vi "LinearSystemId_CreateSingleJointedArmSystem.vi"(9 "G":dbl, 10 "jKgSquaredMeters":dbl, 11 "DCMOTOR":T1 {"Jr_KgM2" format="%13.5p"; "L_H" format="%13.5p"; "Kt_NMPerAmp" format="%13.5p"; "KvINV_RadPerSecPerVolt" format="%13.5p"; "R_Ohms" format="%13.5p"; "FreeSpeed_RadPerSec" format="%13.5p"; "FreeCurrent_Amps" format="%13.5p"; "StallCurrent_Amps" format="%13.5p"; "StallTorque_NM" format="%13.5p"; "nominalVoltage_Volts" format="%13.5p"}) -> (0 "Size Coerced":bool, 3 "Linearsystem":T2)   [LabVIEW 2019, in "Trajectory_Library.lvlib"]
doc: "Create a state-space model of a single jointed arm system. The states of the system are [angle, angular velocity], inputs are [voltage], and outputs are [angle].\n\nInputs: \n - motor -- The motor (or gearbox) attached to the arm.\n - jKgSquaredMeters -- The moment of inertia J of the arm.\n - G -- The gearing between the motor and arm, in output over input. Most of the time this will be greater than 1.\n\nOutputs:\n - LinearSystem -- A LinearSystem representing the given characterized constants.\n - Error -- A boolean indicating an error occured creating the system. A value of TRUE indicates an error."
uses:
  Trajectory_Library.lvlib
  LINEAR_SYSTEM.ctl
  <vilib>/Analysis/Matrix/Datatypes/RealMatrix.ctl
  DCMOTOR.CTL
  <vilib>/Analysis/Matrix/NI_Matrix.lvlib
panel:
  # "<States,States>"
  # "<States,Inputs>"
  # "<Outputs,States>"
  # "<Outputs,Inputs>"
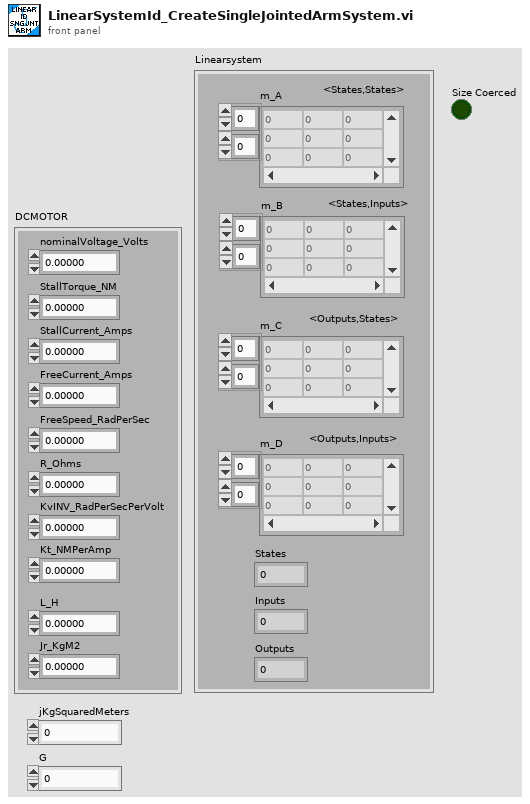
[diagram p1: front panel]
types:
  T1 = typedef "Trajectory_Library.lvlib/DCMOTOR.CTL" = cluster{"nominalVoltage_Volts":dbl, "StallTorque_NM":dbl, "StallCurrent_Amps":dbl, "FreeCurrent_Amps":dbl, "FreeSpeed_RadPerSec":dbl, "R_Ohms":dbl, "KvINV_RadPerSecPerVolt":dbl, "Kt_NMPerAmp":dbl, "L_H":dbl, "Jr_KgM2":dbl}
  T2 = typedef "Trajectory_Library.lvlib/LINEAR_SYSTEM.ctl" = cluster{"m_A":T3, "m_B":T3, "m_C":T3, "m_D":T3, "States":i32, "Inputs":i32, "Outputs":i32}
  T3 = typedef "NI_Matrix.lvlib/RealMatrix.ctl" = dbl[][]
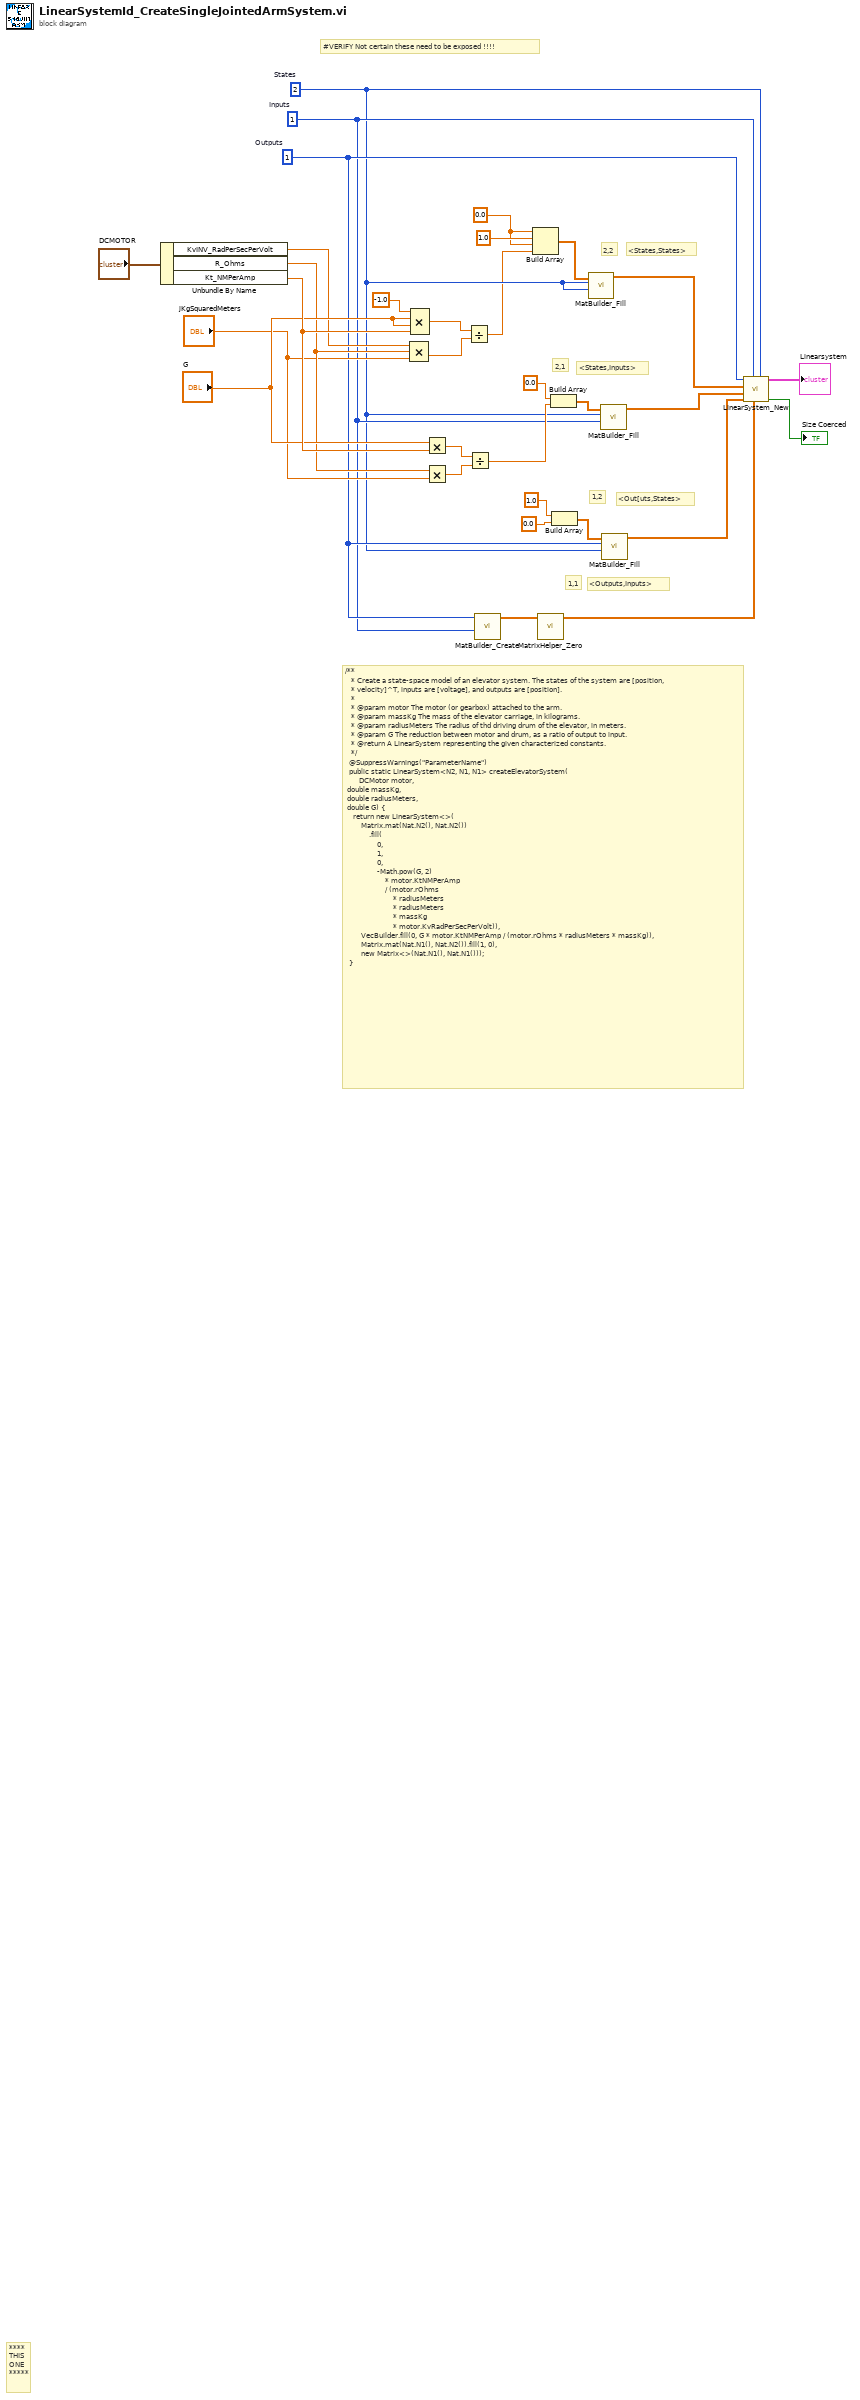
[diagram p0: block diagram]
diagram:
  w16 = 1  # Outputs
  w10 = 1  # Inputs
  w6 = 2  # States
  w4 = 0.0 ("element")
  # "2,2"
  # "2,1"
  # "1,2"
  # "1,1"
  # "<States,States>"
  # "<States,Inputs>"
  # "<Out[uts,States>"
  # "<Outputs,Inputs>"
  # "#VERIFY Not certain these need to be exposed !!!!"
  # "/**\n   * Create a state-space model of an elevator system. The states of the system are [position,\n   * velocity]^T, inputs are [voltage], and outputs are [position].\n   *\n   * @param motor The motor (or gearbox) attached to the arm.\n   * @param massKg The mass of the elevator carriage, in kilograms.\n   * @param radiusMeters The radius of thd driving drum of the elevator, in meters.\n   * @param G The reduction between motor and drum, as a ratio of output to input.\n   * @return A LinearSystem representing the given characterized constants.\n   */\n  @SuppressWarnings(\"ParameterName\")\n  public static LinearSystem<N2, N1, N1> createElevatorSystem(\n      \tDCMotor motor, \n\tdouble massKg, \n\tdouble radiusMeters, \n\tdouble G) {\n    return new LinearSystem<>(\n        Matrix.mat(Nat.N2(), Nat.N2())\n            .fill(\n                0,\n                1,\n                0,\n                -Math.pow(G, 2)\n                    * motor.KtNMPerAmp\n                    / (motor.rOhms\n                        * radiusMeters\n                        * radiusMeters\n                        * massKg\n                        * motor.KvRadPerSecPerVolt)),\n        VecBuilder.fill(0, G * motor.KtNMPerAmp / (motor.rOhms * radiusMeters * massKg)),\n        Matrix.mat(Nat.N1(), Nat.N2()).fill(1, 0),\n        new Matrix<>(Nat.N1(), Nat.N1()));\n  }"
  # "****\nTHIS\nONE\n*****"
  n1 = Unbundle By Name("DCMOTOR") -> ("KvINV_RadPerSecPerVolt"=w22:dbl, "R_Ohms"=w21:dbl, "Kt_NMPerAmp"=w26:dbl)
  n2 = Compound Arithmetic op=MULTIPLY(w22, w21, "jKgSquaredMeters") -> (w27:dbl)
  n3 = Compound Arithmetic op=MULTIPLY(-1.0 ("value"), "G", "G", w26) -> (w28:dbl)
  n4 = Multiply(x="G", y=w26) -> (x*y=w25:dbl)
  n5 = Multiply(x=w21, y="jKgSquaredMeters") -> (x*y=w24:dbl)
  n6 = Divide(x=w28, y=w27) -> (x/y=w3:dbl)
  n7 = Divide(x=w25, y=w24) -> (x/y=w11:dbl)
  n8 = call "MatBuilder_Create.vi"("Columns"=w10, "Rows"=w16) -> ("output matrix"=w9:T3)  [unwired: 9 in]
  n9 = Build Array(w4, 1.0 ("element"), w4, w3) -> (w7:dbl[])
  n10 = call "MatrixHelper_Zero.vi"("input matrix"=w9) -> ("output matrix"=w8:T3)  [unwired: 10 in]
  n11 = Build Array(0.0 ("element"), w11) -> (w13:dbl[])
  n12 = Build Array(1.0 ("element"), 0.0 ("element")) -> (w17:dbl[])
  n13 = call "MatBuilder_Fill.vi"("Columns"=w6, "Rows"=w6, "Value List"=w7) -> ("output matrix"=w2:T3)  [unwired: 8 in]
  n14 = call "MatBuilder_Fill.vi"("Columns"=w10, "Rows"=w6, "Value List"=w13) -> ("output matrix"=w12:T3)  [unwired: 8 in]
  n15 = call "MatBuilder_Fill.vi"("Columns"=w6, "Rows"=w16, "Value List"=w17) -> ("output matrix"=w15:T3)  [unwired: 8 in]
  n16 = call "LinearSystem_New.vi"("States"=w6, "D"=w8, "Inputs"=w10, "C"=w15, "B"=w12, "A"=w2, "Outputs"=w16) -> ("Size Coerced"=→"Size Coerced":bool, "Linearsystem"=→"Linearsystem":T2)  [unwired: 3 in]
